vi "Main.vi"(8 "error in":errorcluster, 11 "subPanel Worker in":refnum<class "subPanel Worker.lvclass">) -> (0 "error out":errorcluster, 3 "subPanel Worker out":refnum<class "subPanel Worker.lvclass">)   [LabVIEW 2017, in "subPanel Worker.lvclass"]
doc: "The <b>Queued Message Handler</b> of the Worker that owns this VI."
uses:
  subPanel Worker.lvclass
  C:/Program Files (x86)/National Instruments/LabVIEW 2017/vi.lib/addons/_Workers/Library/Classes/Worker/Worker.lvclass
  Initialization Data.ctl
  Response Cases.ctl
  subPanel Worker.lvclass/subPanel Worker.ctl
  rql_Set Update Rate.ctl
  rwr_Get Main VI Ref.ctl
  rwr_Get Main VI Ref Reply.ctl
  <vilib>/addons/_Workers/Library/Classes/Message Queue/Message Queue.lvclass
  Message Pump/Message Pump.lvclass
panel:
  in  "Update Rate (ms)":i32=20 min=20
  out "Waveform Chart":dbl(graph)
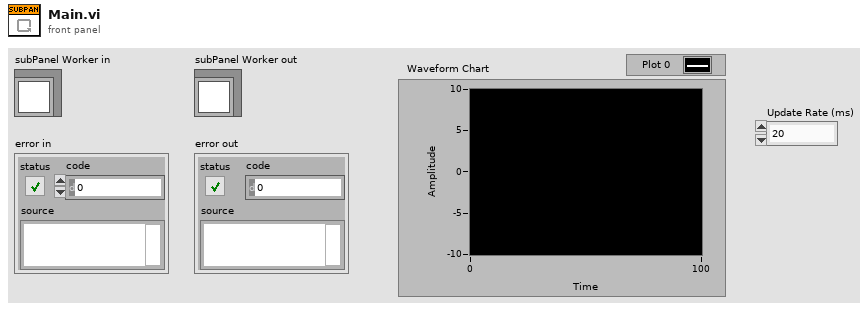
[diagram p1: front panel]
types:
  T1 = typedef "subPanel Worker.lvclass/Initialization Data.ctl" = cluster{"Response Cases":T2}
  T2 = typedef "subPanel Worker.lvclass/Response Cases.ctl" = cluster{"Placeholder - Can be deleted":string}
  T3 = typedef "subPanel Worker.lvclass/rql_Set Update Rate.ctl" = cluster{"String":string}
  T4 = typedef "subPanel Worker.lvclass/rwr_Get Main VI Ref Reply.ctl" = cluster{"VI Ref":refnum<vi>}
  T5 = typedef "subPanel Worker.lvclass/rwr_Get Main VI Ref.ctl" = cluster{"String":string}
  T6 = typedef "Workers.lvlib/Case Label.ctl" = string
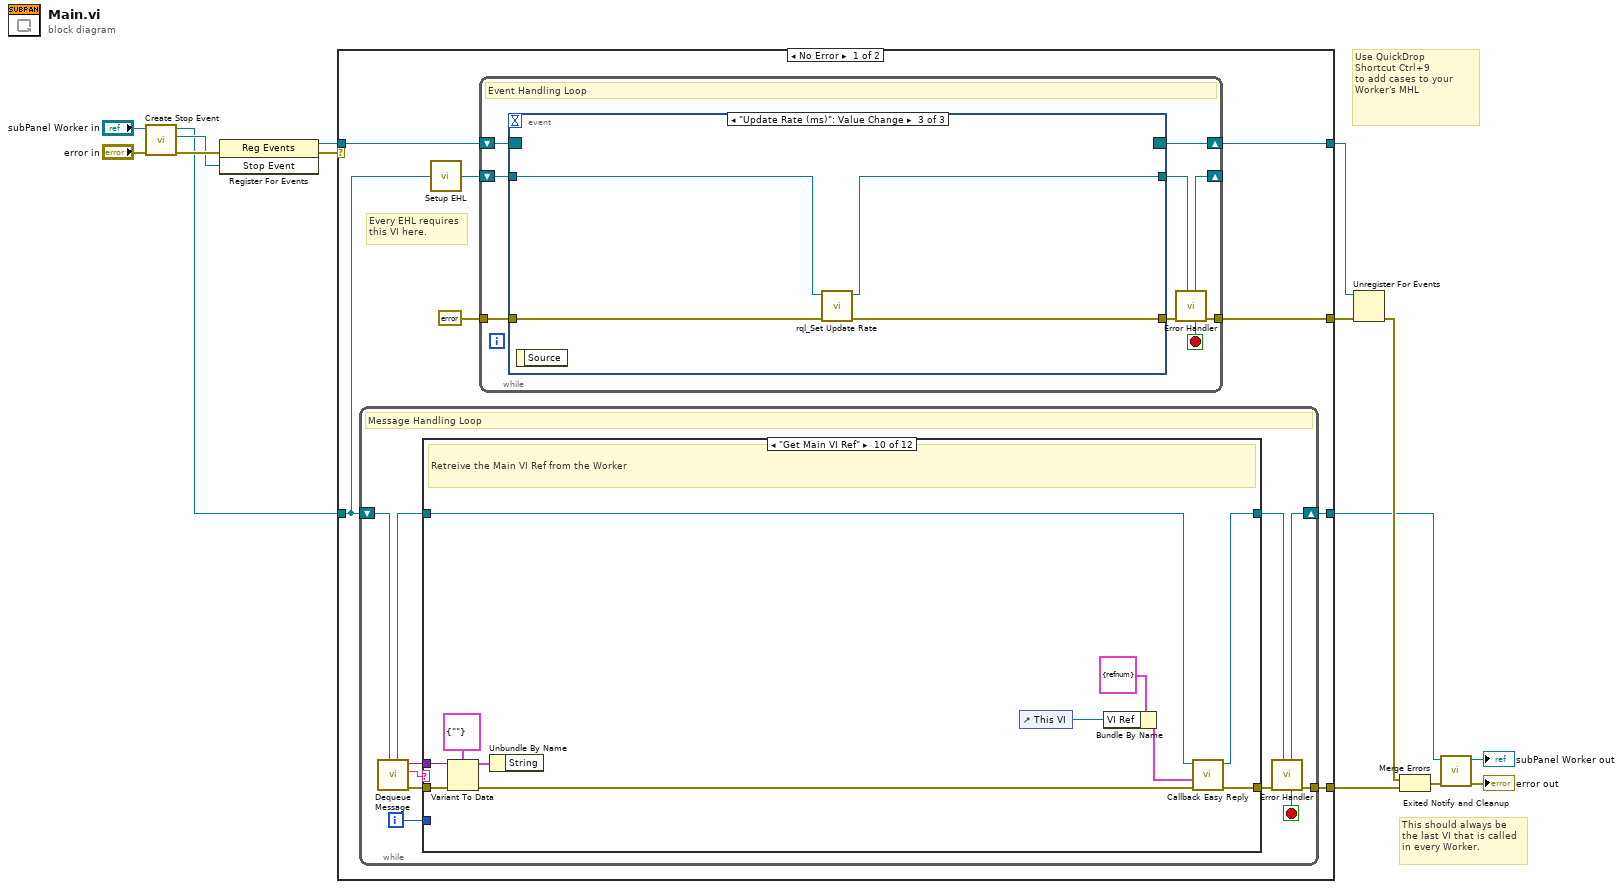
[diagram p0: block diagram]
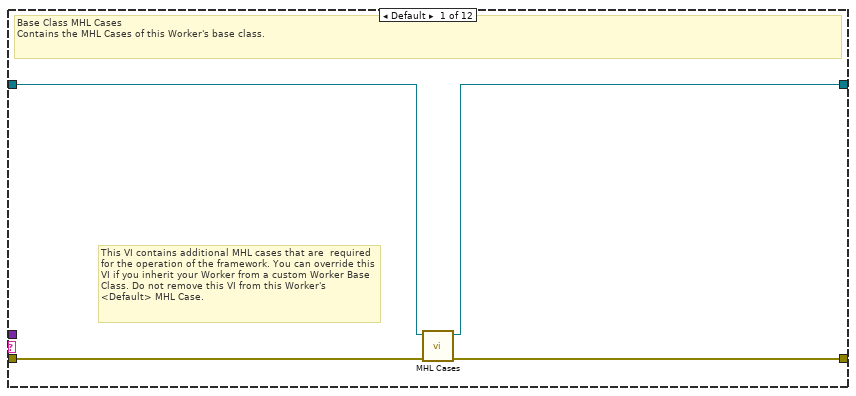
[diagram p2: hidden frame]
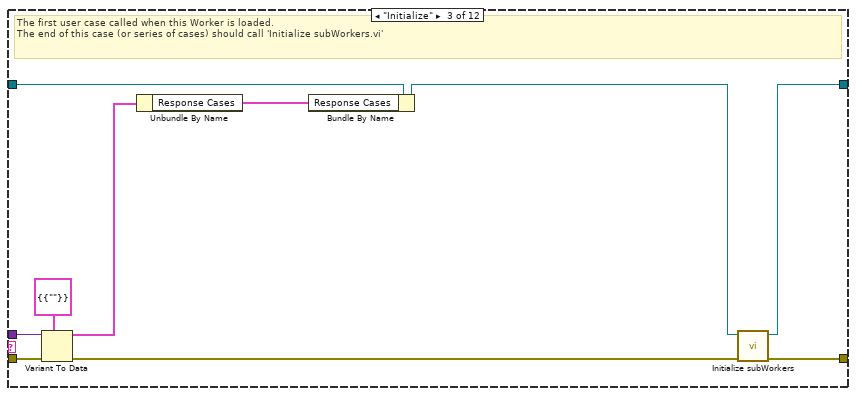
[diagram p4: hidden frame]
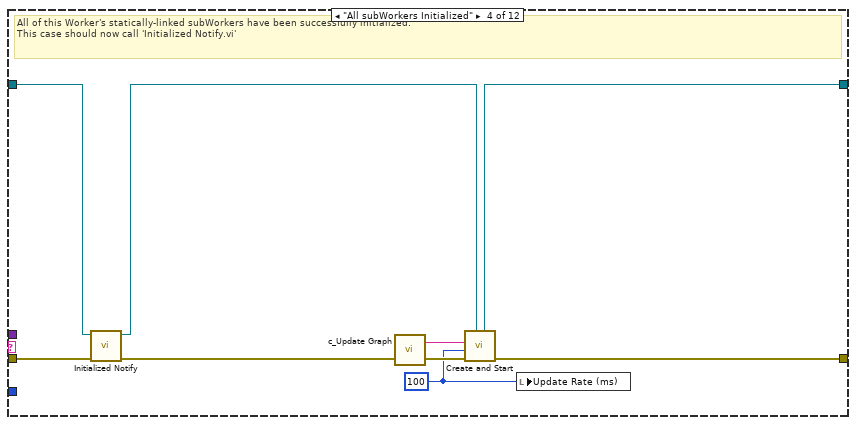
[diagram p5: hidden frame]
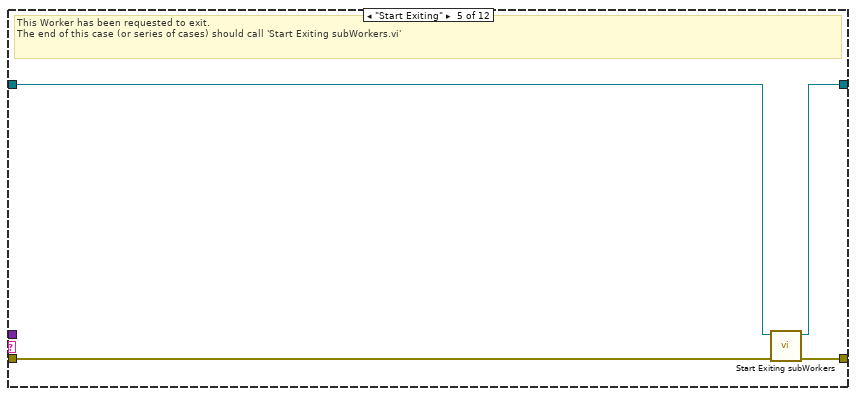
[diagram p6: hidden frame]
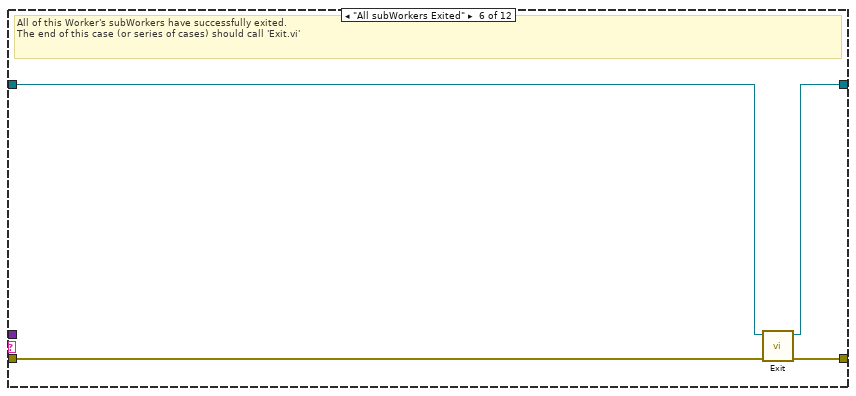
[diagram p7: hidden frame]
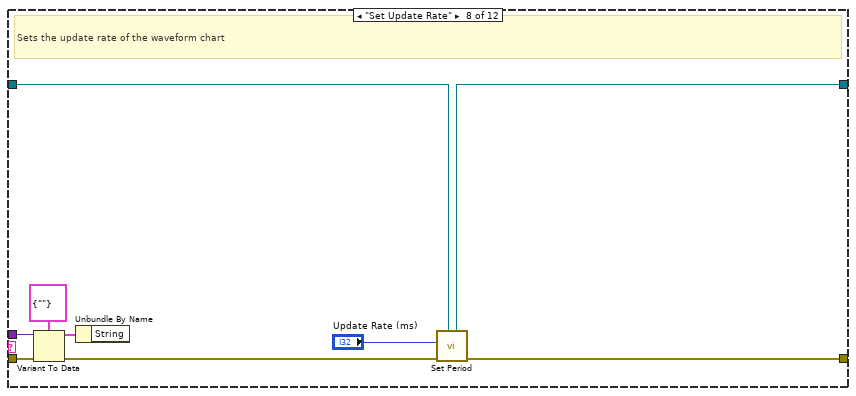
[diagram p9: hidden frame]
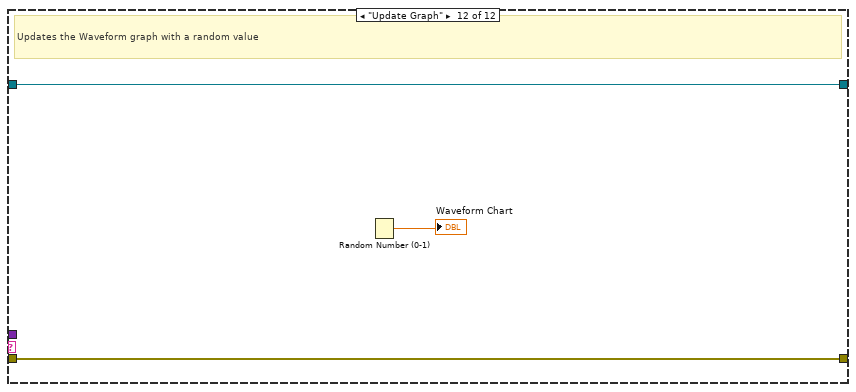
[diagram p12: hidden frame]
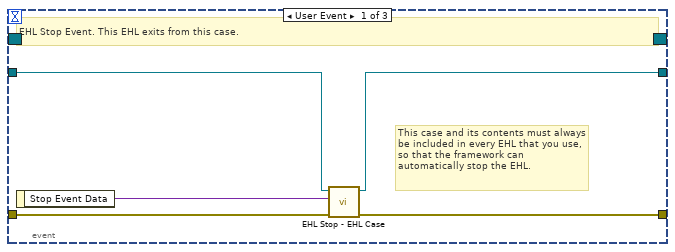
[diagram p13: hidden frame]
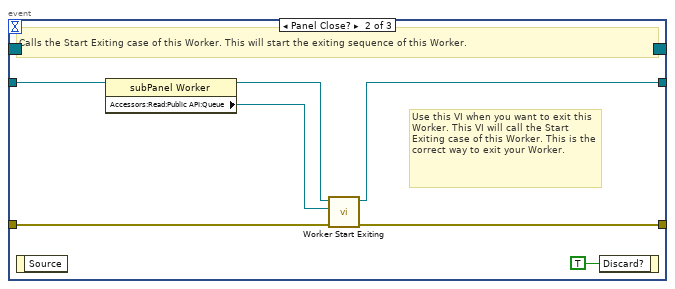
[diagram p14: hidden frame]
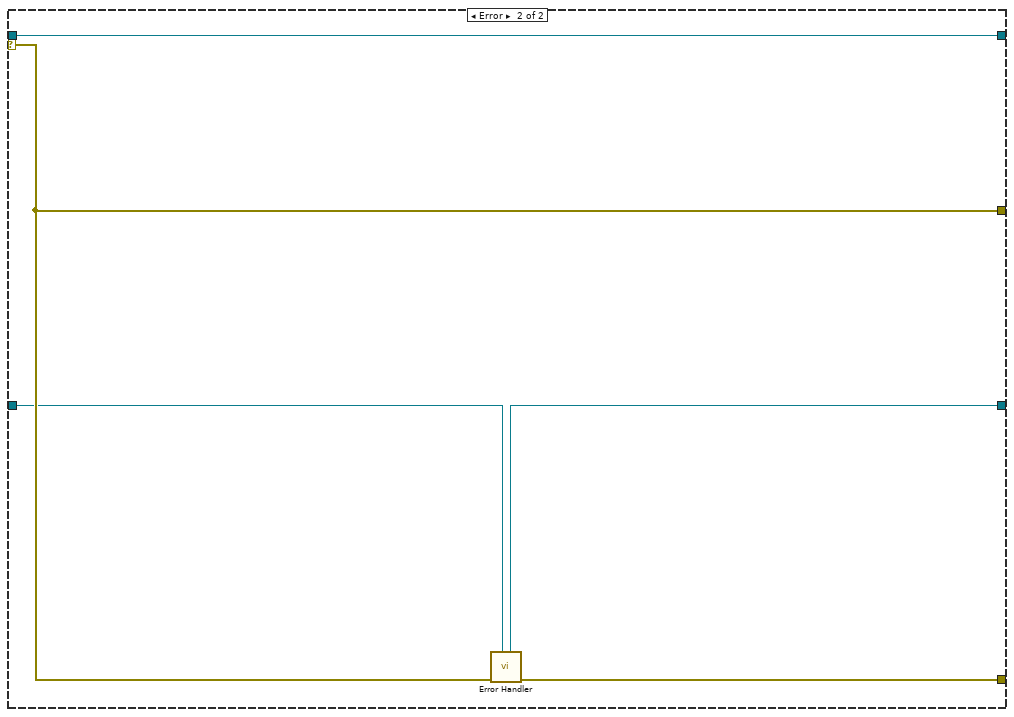
[diagram p15: hidden frame]
diagram:
  # "Use QuickDrop\nShortcut Ctrl+9\nto add cases to your\nWorker's MHL"
  # "This should always be the last VI that is called in every Worker."
  n1 = call-dynamic "Create Stop Event.vi"("error in"="error in", "Worker"="subPanel Worker in") -> ("error out"=w10:errorcluster, "Stop Event"=w7:refnum<user-event>, "Worker out"=w4:refnum<class "subPanel Worker.lvclass">)  [unwired: 7 in]
  n2 = register-events(error in=w10, w7) -> (reference out=w9:refnum<event-registration>, error out=w1:errorcluster)  [unwired: 1 in]
  n3 = case shown="No Error" w1 {
    tunnel: w4 -> [w18 w122]
    tunnel: [w16 w123] -> w8
    tunnel: w9 -> [w23 w124]
    tunnel: [w20 w125] -> w14
    tunnel: [w22 w124] -> w13
    tunnel: [w17 w121] -> w11
    selector: w1 -> [_ w125]
    frame No Error {
      # "Every EHL requires\nthis VI here."
      n4 = while {
        shift-right: [w32] -> w17
        shift-left: w18 -> [w34]
        tunnel: [w33] -> w16
        i -> [w25]
        stop <- w26 stop-if-true
        # "Message Handling Loop"
        n5 = call-dynamic "Dequeue Message.vi"("Worker"=w34) -> ("error out"=w31:errorcluster, "Case out"=w27:string, "Data out"=w24:variant, "Worker out"=w29:refnum<class "subPanel Worker.lvclass">)  [unwired: 6 in, 1 out]
        n6 = case "Worker MHL Case Structure (DO NOT CHANGE LABEL NAME)" shown="\"Get Main VI Ref\"" w27 {
          tunnel: w31 -> [w38 w39 w48 w57 w59 w66 w68 w77 w79 w90 w92 w95]
          tunnel: [w37 w39 w50 w55 w62 w65 w68 w72 w79 w85 w92 w95] -> w30
          tunnel: w29 -> [w36 w40 w47 w58 w60 w64 w67 w71 w78 w83 w91 w94]
          tunnel: [w35 w40 w49 w53 w61 w63 w67 w70 w78 w84 w91 w94] -> w28
          tunnel: w25 -> [_ _ _ _ _ _ _ _ _ _ _ _]
          tunnel: w24 -> [_ _ w45 _ _ _ _ w74 _ w87 _ _]
          frame Default {
            # "This VI contains additional MHL cases that are  required for the operation of the framework. You can override this VI if you inherit your Worker from a custom Worker Base Class. Do not remove this VI from this Worker's <Default> MHL Case."
            # "Base Class MHL Cases\nContains the MHL Cases of this Worker's base class."
            n7 = call-dynamic "MHL Cases.vi"("error in"=w38, "Worker in"=w36) -> ("error out"=w37:errorcluster, "Worker out"=w35:refnum<class "subPanel Worker.lvclass">)  [unwired: 8 in]
          }
          frame "------------ FRAMEWORK CASES -----------" {
            # "Start of Workers Framework Cases"
          }
          frame "Initialize" {
            # "The first user case called when this Worker is loaded.\nThe end of this case (or series of cases) should call 'Initialize subWorkers.vi'"
            n8 = Variant To Data(error in=w48, type=T1 {"Response Cases"={"Placeholder - Can be deleted"=""}} ("Initialization Data"), Variant=w45) -> (data=w43:T1, error out=w46:errorcluster)
            n9 = Unbundle By Name(w43) -> ("Response Cases"=w42:T2)
            n10 = Bundle By Name(cluster=w47, "Response Cases"=w42) -> (w44:refnum<class "subPanel Worker.lvclass">)
            n11 = call-dynamic "Initialize subWorkers.vi"("error in"=w46, "Worker"=w44) -> ("error out"=w50:errorcluster, "dup Worker out"=w49:refnum<class "subPanel Worker.lvclass">)  [unwired: 8 in]
          }
          frame "All subWorkers Initialized" {
            w51 = 100 ("Period (ms)")
            # "All of this Worker's statically-linked subWorkers have been successfully initialized.\nThis case should now call 'Initialized Notify.vi'"
            n12 = call-dynamic "Initialized Notify.vi"("error in"=w57, "Worker"=w58) -> ("error out"=w56:errorcluster, "dup Worker out"=w54:refnum<class "subPanel Worker.lvclass">)  [unwired: 8 in]
            n13 = call "c_Update Graph.vi"() -> ("Case Label"=w52:T6)  [unwired: 1 in]
            n14 = call "Create and Start.vi"("Caller"=w54, "error in (no error)"=w56, "Period (ms)"=w51, "Time Elapsed Response Case (Case Label)"=w52) -> ("error out"=w55:errorcluster, "dup Caller out"=w53:refnum<class "subPanel Worker.lvclass">)  [unwired: 5 in, 1 out]
            n15 = local write "Update Rate (ms)"(w51) -> ()
          }
          frame "Start Exiting" {
            # "This Worker has been requested to exit. \nThe end of this case (or series of cases) should call 'Start Exiting subWorkers.vi'"
            n16 = call-dynamic "Start Exiting subWorkers.vi"("error_in"=w59, "Worker"=w60) -> ("error out"=w62:errorcluster, "dup Worker out"=w61:refnum<class "subPanel Worker.lvclass">)  [unwired: 8 in]
          }
          frame "All subWorkers Exited" {
            # "All of this Worker's subWorkers have successfully exited. \nThe end of this case (or series of cases) should call 'Exit.vi'"
            n17 = call-dynamic "Exit.vi"("error_in"=w66, "Worker"=w64) -> ("error out"=w65:errorcluster, "dup Worker out"=w63:refnum<class "subPanel Worker.lvclass">)  [unwired: 8 in]
          }
          frame "------------- LOCAL API CASES -------------" {
            # "Start of Workers Local API Cases"
          }
          frame "Set Update Rate" {
            # "Sets the update rate of the waveform chart"
            n18 = Variant To Data(error in=w77, type=T3 {"String"=""} ("Data"), Variant=w74) -> (data=w73:T3, error out=w76:errorcluster)
            n19 = Unbundle By Name(w73) -> ()  [unwired: 1 out]
            n20 = call "Set Period.vi"("Caller"=w71, "error in"=w76, "Period (ms)"="Update Rate (ms)") -> ("error out"=w72:errorcluster, "dup Caller out"=w70:refnum<class "subPanel Worker.lvclass">)  [unwired: 7 in]
          }
          frame "------------- PUBLIC API CASES -------------" {
            # "Start of Workers Public API Cases"
          }
          frame "Get Main VI Ref" {
            # "Retreive the Main VI Ref from the Worker"
            n21 = Variant To Data(error in=w90, type=T5 {"String"=""} ("Data"), Variant=w87) -> (data=w86:T5, error out=w89:errorcluster)
            n22 = Unbundle By Name(w86) -> ()  [unwired: 1 out]
            n23 = control-ref of="This VI"() -> (w80:refnum<vi>)
            n24 = Bundle By Name(cluster=T4 {"VI Ref"=refnum} ("Reply Data"), "VI Ref"=w80) -> (w81:T4)
            n25 = call-dynamic "Callback Easy Reply.vi"("error in"=w89, "Data"=w81, "Worker"=w83) -> ("error out"=w85:errorcluster, "dup Worker out"=w84:refnum<class "subPanel Worker.lvclass">)  [unwired: 7 in]
          }
          frame "------------- RESPONSE CASES --------------" {
            # "Start of Workers Response Cases"
          }
          frame "Update Graph" {
            # "Updates the Waveform graph with a random value"
            n26 = Random Number (0-1)() -> (number: 0 to 1=→"Waveform Chart":dbl)
          }
        }
        n27 = call-dynamic "Error Handler.vi"("Worker"=w28, "error_in"=w30) -> ("error out"=w33:errorcluster, "Stop Loop"=w26:bool, "Worker out"=w32:refnum<class "subPanel Worker.lvclass">)  [unwired: 7 in]
      }
      n28 = call-dynamic "Setup EHL.vi"("Worker"=w18) -> ("Worker out"=w19:refnum<class "subPanel Worker.lvclass">)  [unwired: 14 in]
      n29 = while "Event Handling Loop" {
        shift-right: [w104] -> w22
        shift-left: w23 -> [w103]
        tunnel: [w99] -> w20
        tunnel: errorcluster {"status"=FALSE, "code"=0, "source"=""} ("error constant") -> [w101]
        shift-right: [w97] -> _
        shift-left: w19 -> [w102]
        stop <- w96 stop-if-true
        # "Event Handling Loop"
        n30 = event shown="[2] \"Update Rate (ms)\": Value Change" {
          selector: w103 -> [_ _ _]
          dyn-events: [_ _ _] -> w104
          timeout: _ -> [_ _ _]
          tunnel: [w108 w115 w119] -> w100
          tunnel: w101 -> [w109 w114 w120]
          tunnel: w102 -> [w107 w113 w118]
          tunnel: [w106 w112 w117] -> w98
          event User Event {
            # "This case and its contents must always be included in every EHL that you use, so that the framework can automatically stop the EHL."
            # "EHL Stop Event. This EHL exits from this case."
            n31 = event-data() -> ("Stop Event Data"=w105:variant)  [unwired: 1 in]
            n32 = call-dynamic "EHL Stop - EHL Case.vi"("error in"=w109, "Stop Event Data"=w105, "Worker"=w107) -> ("error out"=w108:errorcluster, "Worker out"=w106:refnum<class "subPanel Worker.lvclass">)  [unwired: 7 in]
          }
          event Panel Close? {
            # "Use this VI when you want to exit this Worker. This VI will call the Start Exiting case of this Worker. This is the correct way to exit your Worker."
            # "Calls the Start Exiting case of this Worker. This will start the exiting sequence of this Worker."
            n33 = event-data() -> ()  [unwired: 1 in, 1 out]
            n34 = property class="subPanel Worker"(reference=w113) -> (reference out=w111:refnum<class "subPanel Worker.lvclass">, "Accessors:Read:Public API:Queue"=w110:refnum<class "Message Queue.lvclass">)  [unwired: 1 in, 1 out]
            n35 = call-dynamic "Worker Start Exiting.vi"("error_in"=w114, "Message Queue"=w110, "Worker"=w111) -> ("error out"=w115:errorcluster, "dup Worker out"=w112:refnum<class "subPanel Worker.lvclass">)  [unwired: 7 in]
            n36 = event-data("Discard?"=TRUE) -> ()  [unwired: 1 in, 1 out]
          }
          event "Update Rate (ms)": Value Change {
            n37 = event-data() -> ()  [unwired: 1 in, 1 out]
            n38 = call "rql_Set Update Rate.vi"("error in"=w120, "subPanel Worker in"=w118) -> ("error out"=w119:errorcluster, "dup subPanel Worker out"=w117:refnum<class "subPanel Worker.lvclass">)  [unwired: 8 in]
          }
        }
        n39 = call-dynamic "Error Handler.vi"("Worker"=w98, "error_in"=w100) -> ("error out"=w99:errorcluster, "Stop Loop"=w96:bool, "Worker out"=w97:refnum<class "subPanel Worker.lvclass">)  [unwired: 7 in]
      }
    }
    frame Error {
      n40 = call-dynamic "Error Handler.vi"("Worker"=w122, "error_in"=w125) -> ("error out"=w123:errorcluster, "Worker out"=w121:refnum<class "subPanel Worker.lvclass">)  [unwired: 7 in, 1 out]
    }
  }
  n41 = Unregister For Events(event registration refnum=w13, error in=w14) -> (error out=w15:errorcluster)
  n42 = Merge Errors(w15, w8) -> (w12:errorcluster)
  n43 = call-dynamic "Exited Notify and Cleanup.vi"("error_in"=w12, "Worker"=w11) -> ("error out"=→"error out":errorcluster, "dup Worker out"=→"subPanel Worker out":refnum<class "subPanel Worker.lvclass">)  [unwired: 8 in]
